vi "3_2_PTLF_Classification_Eval(FPGA)(PXI,sbRIO_Remote).vi"() -> ()   [LabVIEW 2020]
doc: "This example demonstrates the usage of \"Deep Neural Network Accelerator for FPGA\" for Face detection and running for inference on RT targets using FPGA."
uses:
  <vilib>/userDefined/High Color/nirio_resource_hc.ctl
  4973630c-52a8-4b5a-885b-d0de098afee9.vi
  0a2e89f5-e3e7-4dda-8136-2185c3411736.vi
  <vilib>/Ngene/Deep Learning Toolkit/Toolkit/NN_Data/subVIs/Get_Data_Vals/2D/NN_Data_Get_ValByRef(2D_SGL).vi
  <vilib>/Ngene/Deep Learning Toolkit/Toolkit/NN_Data/subVIs/Dataset/NN_Variant_to_DVR/2D/NN_Data_Variant_to_DVR(2D_SGL).vi
  <vilib>/FPGAPlugInAG/Dynamic/niLvFpga_Download_Dynamic.vi
  <vilib>/FPGAPlugInAG/Dynamic/niLvFpga_Run_Dynamic.vi
  <vilib>/Ngene/Deep Learning Toolkit/Toolkit/NN_Data/subVIs/Get_Data_Vals/2D/NN_Data_Get_ValByRef(2D_SGL_idx).vi
  <vilib>/Ngene/DeepLTK FPGA Addon/Toolkit/NNF_Host/API/NNF_Set_Input/NNF_Set_Input(1D_I8).vi
  <vilib>/Ngene/Deep Learning Toolkit/Toolkit/NN_Train/Eval_Loss/NN_Eval_Test_Error_Loss/NN_Eval(In1D_Out1D).vi
  <vilib>/Ngene/Deep Learning Toolkit/Toolkit/NN_Train/Eval_Loss/NN_Calc_Cofusion_Matrix/NN_Calc_Confusion_Matrix(In1D_Out1D).vi
  <vilib>/FPGAPlugInAG/Dynamic/niLvFpga_Close_Dynamic.vi
  <vilib>/rvi/interface/nirviMethod/nirviMethod.xnode
  <vilib>/rvi/interface/nirviCloseFPGA/nirviCloseFPGA.xnode
  <vilib>/Ngene/Deep Learning Toolkit/Toolkit/Deep_Learning_Toolkit_by_Ngene.lvlib
  <vilib>/Ngene/DeepLTK FPGA Addon/Toolkit/DeepLTK_FPGA_Addon.lvlib
  <vilib>/ptbypt/NI_PtbyPt.lvlib
panel:
  out "Dataset Size":i32=1200
  in  "FPGA Bitfile":path=path "D:/Ngene/GitHub/deepltk_fpga_examples/FPGA Bitfiles/NNF_sbRIO_9609_8Cores_120MHz.lvbitx"
  in  "FPGA target":T1="rio://10.0.0.39/RIO0" caption="RIO Device"
  out "Loop time(s)":dbl=12.583108442776332 format="%#_4p"
  out "Inference time(s)":dbl=0.07947161899999969 format="%#_4p"
  in  "Stop":bool
  out "Iterations":i32=1199
  in  "Dataset":path=path "D:/Ngene/GitHub/deepltk_fpga_examples/3_PTLF_Classification(PXI,sbRIO)/Dataset/Test"
  in  "Force CPU(All)?":bool
  out "GT":string="Swell"
  out "Pred":string="Sag"
  in  "index":i32=5
  out "Incorectly Classified Sample":sgl[](graph)=[-0.499, -0.502, -0.505, -0.507, -0.509, -0.51, -0.511, -0.512, -0.512, -0.512, -0.511, -0.51, -0.508, -0.506, -0.504, -0.501, -0.498, -0.495, -0.491, -0.487, -0.482, -0.477, -0.471, -0.466, -0.459, -0.453, -0.446, -0.439, -0.431, -0.423, -0.415, -0.406, -0.397, -0.388, -0.378, -0.368, -0.358, -0.347, -0.336, -0.325, -0.314, -0.303, -0.291, -0.279, -0.266, -0.254, -0.241, -0.228, -0.215, -0.202, -0.189, -0.175, -0.161, -0.148, -0.134, -0.12, -0.105, -0.091, -0.077, -0.062, -0.048, -0.034, -0.019, -0.005, 0.01, 0.024, 0.039, 0.053, 0.068, 0.082, 0.096, 0.111, 0.125, 0.139, 0.153, 0.166, 0.18, 0.193, 0.207, 0.22, 0.233, 0.246, 0.258, 0.271, 0.283, 0.295, 0.307, 0.318, 0.329, 0.34, 0.351, 0.362, 0.372, 0.381, 0.391, 0.4, 0.409, 0.418, 0.426, 0.434, 0.441, 0.448, 0.455, 0.462, 0.468, 0.473, 0.479, 0.484, 0.488, 0.492, 0.496, 0.5, 0.502, 0.505, 0.507, 0.509, 0.51, 0.511, 0.512, 0.512, 0.512, 0.511, 0.51, 0.508, 0.506, 0.504, 0.501, 0.498, 0.494, 0.49, 0.486, 0.481, 0.476, 0.471, 0.465, 0.459, 0.452, 0.445, 0.438, 0.43, 0.422, 0.414, 0.405, 0.396, 0.386, 0.377, 0.367, 0.357, 0.346, 0.335, 0.324, 0.313, 0.301, 0.289, 0.277, 0.265, 0.252, 0.24, 0.227, 0.214, 0.2, 0.187, 0.173, 0.16, 0.146, 0.132, 0.118, 0.104, 0.089, 0.075, 0.061, 0.046, 0.032, 0.017, 0.003, -0.012, -0.026, -0.041, -0.055, -0.069, -0.084, -0.098, -0.112, -0.126, -0.14, -0.154, -0.168, -0.182, -0.195, -0.208, -0.222, -0.235, -0.247, -0.26, -0.272, -0.284, -0.296, -0.308, -0.32, -0.331, -0.342, -0.352, -0.363, -0.373, -0.383, -0.392, -0.401, -0.41, -0.419, -0.427, -0.435, -0.442, -0.449, -0.456, -0.462, -0.468, -0.474, -0.479, -0.484, -0.489, -0.493, -0.497, -0.5, -0.503, -0.505, -0.507, -0.509, -0.51, -0.511, -0.512, -0.512, -0.511, -0.511, -0.51, -0.508, -0.506, -0.504, -0.501, -0.498, -0.494, -0.49, -0.486, -0.481, -0.476, -0.47, -0.464, -0.458, -0.451, -0.444, -0.437, -0.429, -0.421, -0.413, -0.404, -0.395, -0.385, -0.376, -0.366, -0.355, -0.345, -0.334, -0.323, -0.311, -0.3, -0.288, -0.276, -0.263, -0.251, -0.238, -0.225, -0.212, -0.199, -0.185, -0.172, -0.158, -0.144, -0.13, -0.116, -0.102, -0.088, -0.073, -0.059, -0.045, -0.03, -0.016, -0.001, 0.013, 0.028, 0.042, 0.057, 0.071, 0.085, 0.1, 0.114, 0.128, 0.142, 0.156, 0.17, 0.183, 0.197, 0.21, 0.223, 0.236, 0.249, 0.261, 0.274, 0.286, 0.298, 0.309, 0.321, 0.332, 0.343, 0.354, 0.364, 0.374, 0.384, 0.393, 0.402, 0.411, 0.42, 0.428, 0.436, 0.443, 0.45, 0.457, 0.463, 0.469, 0.475, 0.48, 0.485, 0.489, 0.493, 0.497, 0.5, 0.503, 0.506, 0.508, 0.509, 0.511, 0.511, 0.512, 0.512, 0.511, 0.511, 0.509, 0.508, 0.506, 0.503, 0.5, 0.497, 0.493, 0.489, 0.485, 0.48, 0.475, 0.469, 0.463, 0.457, 0.45, 0.443, 0.436, 0.428, 0.42, 0.412, 0.403, 0.394, 0.384, 0.374, 0.364, 0.354, 0.343, 0.333, 0.321, 0.31, 0.298, 0.286, 0.274, 0.262, 0.249, 0.237, 0.224, 0.211, 0.197, 0.184, 0.17, 0.156, 0.143, 0.129, 0.115, 0.1, 0.086, 0.072, 0.057, 0.043, 0.028, 0.014, -0.001, -0.015, -0.029, -0.044, -0.058, -0.073, -0.087, -0.101, -0.116, -0.13, -0.144, -0.157, -0.171, -0.185, -0.198, -0.211, -0.225, -0.238, -0.25, -0.263, -0.275, -0.287, -0.299, -0.311, -0.322, -0.333, -0.344, -0.355, -0.365, -0.375, -0.385, -0.394, -0.403, -0.412, -0.421, -0.429, -0.436, -0.444, -0.451, -0.458, -0.464, -0.47, -0.475, -0.481, -0.485, -0.49, -0.494, -0.497, -0.501, -0.503, -0.506, -0.508, -0.509, -0.511, -0.511, -0.512, -0.512, -0.511, -0.51, -0.509, -0.508, -0.505, -0.503, -0.5, -0.497, -0.493, -0.489, -0.484, -0.48, -0.474, -0.469, -0.463, -0.456, -0.45, -0.442, -0.435, -0.427, -0.419, -0.41, -0.402, -0.393, -0.383, -0.373, -0.363, -0.353, -0.342, -0.331, -0.32, -0.309, -0.297, -0.285, -0.273, -0.261, -0.248, -0.235, -0.222, -0.209, -0.196, -0.182, -0.169, -0.155, -0.141, -0.127, -0.113, -0.099, -0.084, -0.07, -0.056, -0.041, -0.027, -0.012, 0.002, 0.017, 0.031, 0.046, 0.06, 0.074, 0.089, 0.103, 0.117, 0.131, 0.145, 0.159, 0.173, 0.186, 0.2, 0.213, 0.226, 0.239, 0.252, 0.264, 0.277, 0.289, 0.301, 0.312, 0.324, 0.335, 0.345, 0.356, 0.366, 0.376, 0.386, 0.395, 0.404, 0.413, 0.422, 0.43, 0.437, 0.445, 0.452, 0.458, 0.465, 0.47, 0.476, 0.481, 0.486, 0.49, 0.494, 0.498, 0.501, 0.504, 0.506, 0.508, 0.51, 0.511, 0.511, 0.512, 0.512, 0.511, 0.51, 0.509, 0.507, 0.505, 0.503, 0.5, 0.496, 0.493, 0.488, 0.484, 0.479, 0.474, 0.468, 0.462, 0.456, 0.449, 0.442, 0.434, 0.426, 0.418, 0.409, 0.401, 0.391, 0.382, 0.372, 0.362, 0.352, 0.341, 0.33, 0.319, 0.307, 0.296, 0.284, 0.271, 0.259, 0.246, 0.234, 0.221, 0.207, 0.194, 0.181, 0.167, 0.153, 0.139, 0.125, 0.111, 0.097, 0.083, 0.068, 0.054, 0.04, 0.025, 0.011, -0.004, -0.018, -0.033, -0.047, -0.062, -0.076, -0.09, -0.105, -0.119, -0.133, -0.147, -0.161, -0.174, -0.188, -0.201, -0.215, -0.228, -0.241, -0.253, -0.266, -0.278, -0.29, -0.302, -0.314, -0.325, -0.336, -0.347, -0.357, -0.368, -0.377, -0.387, -0.396, -0.405, -0.414, -0.422, -0.431, -0.438, -0.445, -0.452, -0.459, -0.465, -0.471, -0.477, -0.482, -0.486, -0.491, -0.495, -0.498, -0.501, -0.504, -0.506, -0.508, -0.51, -0.511, -0.512, -0.512, -0.512, -0.511, -0.51, -0.509, -0.507, -0.505, -0.502, -0.499, -0.496, -0.492, -0.488, -0.483, -0.478, -0.473, -0.467, -0.461, -0.455, -0.448, -0.441, -0.433, -0.425, -0.417, -0.408, -0.4, -0.39, -0.381, -0.371, -0.361, -0.35, -0.34, -0.329, -0.317, -0.306, -0.294, -0.282, -0.27, -0.258, -0.245, -0.232, -0.219, -0.206, -0.193, -0.179, -0.165, -0.152, -0.138, -0.124, -0.11, -0.095, -0.081, -0.067, -0.052, -0.038, -0.023, -0.009, 0.006, 0.02, 0.035, 0.049, 0.063, 0.078, 0.092, 0.106, 0.121, 0.135, 0.148, 0.162, 0.176, 0.19, 0.203, 0.216, 0.229, 0.242, 0.255, 0.267, 0.279, 0.292, 0.303, 0.315, 0.326, 0.337, 0.348, 0.359, 0.369, 0.379, 0.388, 0.398, 0.406, 0.415, 0.423, 0.431, 0.439, 0.446, 0.453, 0.46, 0.466, 0.472, 0.477, 0.482, 0.487, 0.491, 0.495, 0.499, 0.502, 0.504, 0.507, 0.508, 0.51, 0.511, 0.512, 0.512, 0.512, 0.511, 0.51, 0.509, 0.507, 0.505, 0.502, 0.499, 0.495, 0.492, 0.487, 0.483, 0.478, 0.472, 0.467, 0.46, 0.454, 0.447, 0.44, 0.432, 0.424, 0.416, 0.407, 0.398, 0.389, 0.38, 0.37, 0.36, 0.349, 0.338, 0.327, 0.316, 0.305, 0.293, 0.281, 0.269, 0.256, 0.243, 0.231, 0.218, 0.204, 0.191, 0.177, 0.164, 0.15, 0.136, 0.122, 0.108, 0.094, 0.079, 0.065, 0.051, 0.036, 0.022, 0.007, -0.007, -0.022, -0.036, -0.051, -0.065, -0.08, -0.094, -0.108, -0.122, -0.136, -0.15, -0.164, -0.178, -0.191, -0.204, -0.218, -0.231, -0.244, -0.256, -0.269, -0.281, -0.293, -0.305, -0.316, -0.328, -0.339, -0.349, -0.36, -0.37, -0.38, -0.389, -0.399, -0.408, -0.416, -0.424, -0.432, -0.44, -0.447, -0.454, -0.461, -0.467, -0.472, -0.478, -0.483, -0.487, -0.492, -0.496, -0.499, -0.502, -0.505, -0.507, -0.509, -0.51, -0.511, -0.512, -0.512, -0.512, -0.511, -0.51, -0.508, -0.507, -0.504, -0.502, -0.499, -0.495, -0.491, -0.487, -0.482, -0.477, -0.472, -0.466, -0.46, -0.453, -0.446, -0.439, -0.431, -0.423, -0.415, -0.406, -0.397, -0.388, -0.378, -0.369, -0.358, -0.348, -0.337, -0.326, -0.315, -0.303, -0.291, -0.279, -0.267, -0.255, -0.242, -0.229, -0.216, -0.203, -0.189, -0.176, -0.162, -0.148, -0.134, -0.12, -0.106, -0.092, -0.078, -0.063, -0.049, -0.034, -0.02, -0.005, 0.009, 0.024, 0.038, 0.052, 0.067, 0.081, 0.095, 0.11, 0.124, 0.138, 0.152, 0.166, 0.179, 0.193, 0.206, 0.219, 0.232, 0.245, 0.258, 0.27, 0.282, 0.294, 0.306, 0.318, 0.329, 0.34, 0.351, 0.361, 0.371, 0.381, 0.39, 0.4, 0.409, 0.417, 0.425, 0.433, 0.441, 0.448, 0.455, 0.461, 0.467, 0.473, 0.478, 0.483, 0.488, 0.492, 0.496, 0.499, 0.502, 0.505, 0.507, 0.509, 0.51, 0.511, 0.512, 0.512, 0.512, 0.511, 0.51, 0.508, 0.506, 0.504, 0.501, 0.498, 0.495, 0.491, 0.486, 0.482, 0.477, 0.471, 0.465, 0.459, 0.452, 0.445, 0.438, 0.43, 0.422, 0.414, 0.405, 0.396, 0.387, 0.377, 0.367, 0.357, 0.347, 0.336, 0.325, 0.313, 0.302, 0.29, 0.278, 0.266, 0.253, 0.24, 0.228, 0.214, 0.201, 0.188, 0.174, 0.161, 0.147, 0.133, 0.119, 0.105, 0.09, 0.076, 0.062, 0.047, 0.033, 0.018, 0.004, -0.011, -0.025, -0.04, -0.054, -0.069, -0.083, -0.097, -0.111, -0.125, -0.139, -0.153, -0.167, -0.181, -0.194, -0.208, -0.221, -0.234, -0.247, -0.259, -0.272, -0.284, -0.296, -0.307, -0.319, -0.33, -0.341, -0.352, -0.362, -0.372, -0.382, -0.392, -0.401, -0.41, -0.418, -0.426, -0.434, -0.442, -0.449, -0.456, -0.462, -0.468, -0.474, -0.479, -0.484, -0.488, -0.493, -0.496, -0.5, -0.503, -0.505, -0.507, -0.509, -0.51, -0.511, -0.512, -0.512, -0.511, -0.511, -0.51, -0.508, -0.506, -0.504, -0.501, -0.498, -0.494, -0.49, -0.486, -0.481, -0.476, -0.47, -0.464, -0.458, -0.452, -0.445, -0.437, -0.429, -0.421, -0.413, -0.404, -0.395, -0.386, -0.376, -0.366, -0.356, -0.345, -0.335, -0.323, -0.312, -0.3, -0.289, -0.276, -0.264, -0.252, -0.239, -0.226, -0.213, -0.2, -0.186, -0.173, -0.159, -0.145, -0.131, -0.117, -0.103, -0.089, -0.074, -0.06, -0.045, -0.031, -0.017, -0.002, 0.012, 0.027, 0.041, 0.056, 0.07, 0.085, 0.099, 0.113, 0.127, 0.141, 0.155, 0.169, 0.182, 0.196, 0.209, 0.222, 0.235, 0.248, 0.261, 0.273, 0.285, 0.297, 0.309, 0.32, 0.331, 0.342, 0.353, 0.363, 0.373, 0.383, 0.393, 0.402, 0.411, 0.419, 0.427, 0.435, 0.443, 0.45, 0.456, 0.463, 0.469, 0.474, 0.48, 0.485, 0.489, 0.493, 0.497, 0.5, 0.503, 0.505, 0.508, 0.509, 0.51, 0.511, 0.512, 0.512, 0.511, 0.511, 0.509, 0.508, 0.693, 0.69, 0.686, 0.682, 0.677, 0.671, 0.665, 0.659, 0.652, 0.644, 0.636, 0.627, 0.618, 0.608, 0.598, 0.588, 0.576, 0.565, 0.553, 0.54, 0.527, 0.514, 0.5, 0.486, 0.472, 0.457, 0.442, 0.426, 0.41, 0.394, 0.377, 0.36, 0.343, 0.325, 0.308, 0.29, 0.272, 0.253, 0.234, 0.216, 0.197, 0.177, 0.158, 0.139, 0.119, 0.1, 0.08, 0.06, 0.04, 0.02, 0.0, -0.019, -0.039, -0.059, -0.079, -0.099, -0.118, -0.138, -0.157, -0.177, -0.196, -0.215, -0.234, -0.252, -0.271, -0.289, -0.307, -0.325, -0.342, -0.359, -0.376, -0.393, -0.409, -0.425, -0.441, -0.456, -0.471, -0.486, -0.5, -0.514, -0.527, -0.54, -0.552, -0.564, -0.576, -0.587, -0.598, -0.608, -0.618, -0.627, -0.635, -0.644, -0.651, -0.658, -0.665, -0.671, -0.677, -0.682, -0.686, -0.69, -0.693, -0.696, -0.698, -0.7, -0.701, -0.702, -0.702, -0.701, -0.7, -0.698, -0.696, -0.693, -0.69, -0.686, -0.681, -0.676, -0.671, -0.665, -0.658, -0.651, -0.643, -0.635, -0.626, -0.617, -0.607, -0.597, -0.586, -0.575, -0.563, -0.551, -0.539, -0.526, -0.513, -0.499, -0.485, -0.47, -0.455, -0.44, -0.424, -0.408, -0.392, -0.375, -0.358, -0.341, -0.323, -0.306, -0.288, -0.269, -0.251, -0.232, -0.213, -0.194, -0.175, -0.156, -0.136, -0.117, -0.097, -0.077, -0.058, -0.038, -0.018, 0.002, 0.022, 0.042, 0.061, 0.081, 0.101, 0.121, 0.14, 0.16, 0.179, 0.198, 0.217, 0.236, 0.254, 0.273, 0.291, 0.309, 0.327, 0.344, 0.361, 0.378, 0.395, 0.411, 0.427, 0.443, 0.458, 0.473, 0.487, 0.501, 0.515, 0.528, 0.541, 0.554, 0.566, 0.577, 0.588, 0.599, 0.609, 0.619, 0.628, 0.464, 0.47, 0.476, 0.481, 0.486, 0.49, 0.494, 0.498, 0.501, 0.504, 0.506, 0.508, 0.51, 0.511, 0.511, 0.512, 0.512, 0.511, 0.51, 0.509, 0.507, 0.505, 0.503, 0.5, 0.497, 0.493, 0.489, 0.484, 0.479, 0.474, 0.468, 0.462, 0.456, 0.449, 0.442, 0.435, 0.427, 0.418, 0.41, 0.401, 0.392, 0.382, 0.373, 0.363, 0.352, 0.342, 0.331, 0.319, 0.308, 0.296, 0.284, 0.272, 0.26, 0.247, 0.234, 0.221, 0.208, 0.195, 0.181, 0.168, 0.154, 0.14, 0.126, 0.112, 0.098, 0.084, 0.069, 0.055, 0.04, 0.026, 0.011, -0.003, -0.018, -0.032, -0.047, -0.061, -0.075, -0.09, -0.104, -0.118, -0.132, -0.146, -0.16, -0.174, -0.187, -0.201, -0.214, -0.227, -0.24, -0.253, -0.265, -0.277, -0.289, -0.301, -0.313, -0.324, -0.335, -0.346, -0.357, -0.367, -0.377, -0.387, -0.396, -0.405, -0.414, -0.422, -0.43, -0.438, -0.445, -0.452, -0.459, -0.465, -0.471, -0.476, -0.481, -0.486, -0.49, -0.494, -0.498, -0.501, -0.504, -0.506, -0.508, -0.51, -0.511, -0.512, -0.512, -0.512, -0.511, -0.51, -0.509, -0.507, -0.505, -0.502, -0.499, -0.496, -0.492, -0.488, -0.484, -0.479, -0.473, -0.468, -0.462, -0.455, -0.448, -0.441, -0.434, -0.426, -0.417, -0.409, -0.4, -0.391, -0.381, -0.372, -0.361, -0.351, -0.34, -0.329, -0.318, -0.307, -0.295, -0.283, -0.271, -0.258, -0.246, -0.233, -0.22, -0.207, -0.193, -0.18, -0.166, -0.152, -0.138, -0.124, -0.11, -0.096, -0.082, -0.068, -0.053, -0.039, -0.024, -0.01, 0.005, 0.019, 0.034, 0.048, 0.063, 0.077, 0.091, 0.106, 0.12, 0.134, 0.148, 0.162, 0.175, 0.189, 0.202, 0.215, 0.228, 0.241, 0.254, 0.267, 0.279, 0.291, 0.303, 0.314, 0.326, 0.337, 0.347, 0.358, 0.368, 0.378, 0.388, 0.397, 0.406, 0.415, 0.423, 0.431, 0.439, 0.446, 0.453, 0.459, 0.466, 0.471, 0.477, 0.482, 0.487, 0.491, 0.495, 0.498, 0.501, 0.504, 0.506, 0.508, 0.51, 0.511, 0.512, 0.512, 0.512, 0.511, 0.51, 0.509, 0.507, 0.505, 0.502, 0.499, 0.496, 0.492, 0.488, 0.483, 0.478, 0.473, 0.467, 0.461, 0.454, 0.447, 0.44, 0.433, 0.425, 0.417, 0.408, 0.399, 0.39, 0.38, 0.37, 0.36, 0.35, 0.339, 0.328, 0.317, 0.305, 0.293, 0.281, 0.269, 0.257, 0.244, 0.231, 0.218, 0.205, 0.192, 0.178, 0.165, 0.151, 0.137, 0.123, 0.109, 0.094, 0.08, 0.066, 0.051, 0.037, 0.022, 0.008, -0.007, -0.021, -0.035, -0.05, -0.064, -0.079, -0.093, -0.107, -0.121, -0.135, -0.149, -0.163, -0.177, -0.19, -0.204, -0.217, -0.23, -0.243, -0.256, -0.268, -0.28, -0.292, -0.304, -0.316, -0.327, -0.338, -0.349, -0.359, -0.369, -0.379, -0.389, -0.398, -0.407, -0.416, -0.424, -0.432, -0.44, -0.447, -0.454, -0.46, -0.466, -0.472, -0.478, -0.483, -0.487, -0.491, -0.495, -0.499, -0.502, -0.504, -0.507, -0.509, -0.51, -0.511, -0.512, -0.512, -0.512, -0.511, -0.51, -0.509, -0.507, -0.504, -0.502, -0.499, -0.495, -0.491, -0.487, -0.482, -0.477, -0.472, -0.466, -0.46, -0.454, -0.447, -0.439, -0.432, -0.424, -0.416, -0.407, -0.398, -0.389, -0.379, -0.369, -0.359, -0.348, -0.338, -0.327, -0.315, -0.304, -0.292, -0.28, -0.268, -0.255, -0.243, -0.23, -0.217, -0.204, -0.19, -0.177, -0.163, -0.149, -0.135, -0.121, -0.107, -0.093, -0.078, -0.064, -0.05, -0.035, -0.021, -0.006, 0.008, 0.023, 0.037, 0.052, 0.066, 0.08, 0.095, 0.109, 0.123, 0.137, 0.151, 0.165, 0.178, 0.192, 0.205, 0.219, 0.232, 0.244, 0.257, 0.269, 0.282, 0.294, 0.305, 0.317, 0.328, 0.339, 0.35, 0.36, 0.37, 0.38, 0.39, 0.399, 0.408, 0.417, 0.425, 0.433, 0.44, 0.448, 0.454, 0.461, 0.467, 0.473, 0.478, 0.483, 0.488, 0.492, 0.496, 0.499, 0.502, 0.505, 0.507, 0.509, 0.51, 0.511, 0.512, 0.512, 0.512, 0.511, 0.51, 0.508, 0.506, 0.504, 0.501, 0.498, 0.495, 0.491, 0.487, 0.482, 0.477, 0.471, 0.466, 0.459, 0.453, 0.446, 0.439, 0.431, 0.423, 0.415, 0.406, 0.397, 0.388, 0.378, 0.368, 0.358, 0.347, 0.336, 0.325, 0.314, 0.302, 0.291, 0.279, 0.266, 0.254, 0.241, 0.228, 0.215, 0.202, 0.189, 0.175, 0.161, 0.147, 0.134, 0.119, 0.105, 0.091, 0.077, 0.062, 0.048, 0.034, 0.019, 0.005, -0.01, -0.024, -0.039, -0.053, -0.068, -0.082, -0.096, -0.111, -0.125, -0.139, -0.153, -0.166, -0.18, -0.194, -0.207, -0.22, -0.233, -0.246, -0.258, -0.271, -0.283, -0.295, -0.307, -0.318, -0.329, -0.34, -0.351, -0.362, -0.372, -0.381, -0.391, -0.4, -0.409, -0.418, -0.426, -0.434, -0.441, -0.448, -0.455, -0.462, -0.468, -0.473, -0.479, -0.484, -0.488, -0.492, -0.496, -0.5, -0.502, -0.505, -0.507]
  out "Confusion Matrix (Table)":string[][](table)=[["200", "0", "0", "0", "0", "0", "1.0000"], ["0", "199", "0", "1", "0", "0", "0.9950"], ["0", "0", "200", "0", "0", "0", "1.0000"], ["0", "0", "0", "200", "0", "0", "1.0000"], ["0", "0", "1", "18", "181", "0", "0.9050"], ["0", "0", "2", "2", "3", "193", "0.9650"], ["1.0000", "1.0000", "0.9852", "0.9050", "0.9837", "1.0000", ""]]
  out "Error":sgl=0.0225
  out "Loss":sgl=0.029398046
  in  "Weight File Path":path=path "D:/Ngene/GitHub/deepltk_fpga_examples/3_PTLF_Classification(PXI,sbRIO)/Models/1_PTLF_Classification_Converted/NNF_ptlf_classifier_weights_24_11_21__13_54_07.bin"
  in  "Configuration File Path":path=path "D:/Ngene/GitHub/deepltk_fpga_examples/3_PTLF_Classification(PXI,sbRIO)/Models/1_PTLF_Classification_Converted/NNF_ptlf_classifier_net_cfg_24_11_21__13_54_07.cfg"
  in  "Scalers File Path":path=path "D:/Ngene/GitHub/deepltk_fpga_examples/3_PTLF_Classification(PXI,sbRIO)/Models/1_PTLF_Classification_Converted/NNF_ptlf_classifier_net_scalers_24_11_21__13_54_07.cfg"
  # "Overview: This VI is designed to evaluate (measure the accuracy of) the model when executed on FPGA in PXI systems.\nThis VI can also be used to run the evaluation on sbRIO Targets remotely (from Windows based PC)\nRequirements: \n• DeepLTK - Deep Learning Toolkit for LabVIEW (https://www.ngene.co/deep-learning-toolkit-for-labview)\n• DeepLTK FPGA Addon (https://www.ngene.co/deepltk-accelerator-for-fpga)\nInstructions:\n1. Select FPGA target at FPGA Target control. PXI or remote sbRIO FPGA target can be specified.\n2. Provide path to compiled FPGA bitfile at FPGA Bitfile control. A sample is available in the \"Examples\\FPGA Bitfiles\" folder. \n3. Provide the path to the dataset to be evaluated at Dataset.\n4. Provide paths to .cfg, .bin and scalers.cfg files generated during model conversion or sample from project (locted in \"Models\\1_PTLF_Classification_Converted\" folder ) at Network Configuration File Path, Weight File Path and Scalers File Path controls.\n5. Run the VI with the default remaining settings.\n6. Observe mersured accuracy at Loss, Error and Confusion Matrix indicators, and analyze Incorectly Classified Sample by selecting samples with help of index control.\n7. Press the Stop button to stop the VI.\n8. To measure reference accuracy (when executed on CPU) run 3_1_PTLF_Classification_Eval(CPU).vi located in the project.\nMore Examples: https://github.com/ngenehub/deepltk_fpga_examples"
  # "Copy resource path from NI MAX if needed"
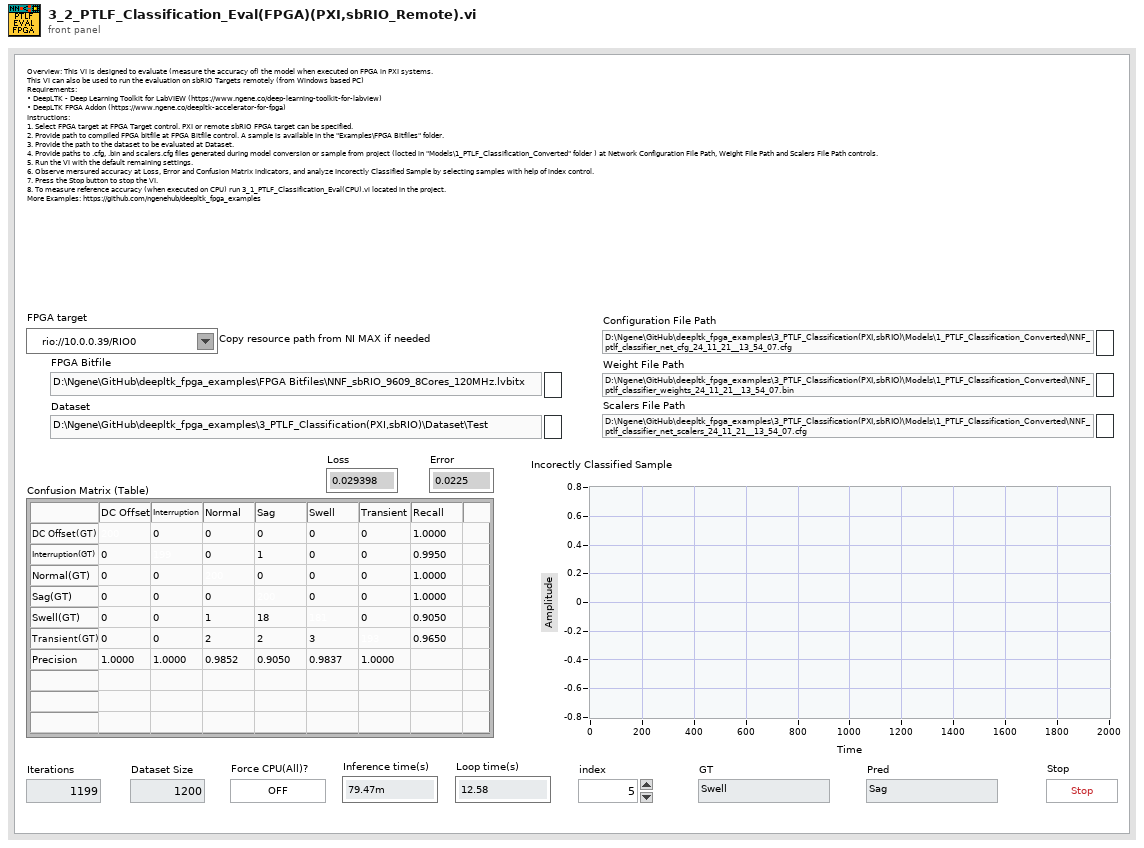
[diagram p1: front panel]
types:
  T1 = typedef "nirio_resource_hc.ctl" = tag
  T2 = typedef "Deep_Learning_Toolkit_by_Ngene.lvlib/NN_DataSets_All(In1D_Out1D).ctl" = cluster{"Train":T3, "Validation":T3, "Test":T3}
  T3 = typedef "Deep_Learning_Toolkit_by_Ngene.lvlib/NN_DataSet(In1D_Out1D).ctl" = cluster{"Inputs Ref.":variant, "Outputs Ref.":T4, "Dims_In":i32, "Dataset_Size":i32, "Dims_Out":i32, "Labels":string[], "File Paths":path[]}
  T4 = typedef "Deep_Learning_Toolkit_by_Ngene.lvlib/NN_Data_ref(2D_SGL).ctl" = refnum<data-value>
  T5 = typedef "DeepLTK_FPGA_Addon.lvlib/NNF.ctl" = cluster{"FPGA VI Ref ":refnum<k20>, "Subnets":T6[], "Dims_In":T8, "#Cores(enum)":T9, "NN_Ref":T10}
  T6 = typedef "DeepLTK_FPGA_Addon.lvlib/NNF_Subnet.ctl" = cluster{"Subnet Type":T7, "Subnet Data":variant, "Input Scaler":sgl, "Output Scaler":sgl}
  T7 = typedef "DeepLTK_FPGA_Addon.lvlib/NNF_Subnet_Type.ctl" = enum16{"CPU", "FPGA", "Split FPGA"}
  T8 = typedef "Deep_Learning_Toolkit_by_Ngene.lvlib/NN_Dims(C,H,W).ctl" = cluster{"C":i32, "H":i32, "W":i32}
  T9 = typedef "DeepLTK_FPGA_Addon.lvlib/NNF_No_Of_Cores.ctl" = enum16{"4CH", "8CH"}
  T10 = typedef "DeepLTK_FPGA_Addon.lvlib/NN_DVR.ctl" = refnum<data-value>
  T11 = typedef "Deep_Learning_Toolkit_by_Ngene.lvlib/NN_Layer.ctl" = cluster{"Name":string, "Layer_Data":variant, "Layer_Type":T12, "Dims_In":T8, "Layers_In":variant, "Dims_Out":T8, "Layers_Out":variant, "Metrics":T13, "GPU_Data":variant, "mBatch":i32, "NN_Device":T14, "NNg_hdls":T15, "Train?":bool, "Dimty":T16, "RecptField":T17}
  T12 = typedef "Deep_Learning_Toolkit_by_Ngene.lvlib/NN_Layer_Type.ctl" = enum16{"Input1D", "Input3D", "Conv1D", "Conv2D", "Conv2D_Adv", "MaxPool", "AvgPool", "UpSample", "DropOut3D", "ShortCut", "Concat", "SoftMax3D", "FC", "DropOut", "Softmax", "Flatten", "YOLO_v2", "YOLO_v4", "Activation", "BatchNormalization", "Unsupported"}
  T13 = typedef "Deep_Learning_Toolkit_by_Ngene.lvlib/NN_Layer_Metrics.ctl" = cluster{"Data":dbl, "Params":dbl, "Ops":dbl}
  T14 = typedef "Deep_Learning_Toolkit_by_Ngene.lvlib/NN_Device.ctl" = enum16{"CPU", "GPU"}
  T15 = typedef "Deep_Learning_Toolkit_by_Ngene.lvlib/nng_cuda_handles.ctl" = cluster{"cudnn":u64, "cublas":u64, "stream":u64, "curand":u64}
  T16 = typedef "Deep_Learning_Toolkit_by_Ngene.lvlib/NN_Layer_Dimty.ctl" = enum16{"1D", "3D"}
  T17 = typedef "Deep_Learning_Toolkit_by_Ngene.lvlib/NN_Layer_RF_State.ctl" = cluster{"Dims":T18, "J":T18}
  T18 = typedef "Deep_Learning_Toolkit_by_Ngene.lvlib/NN_Dims(V,H).ctl" = cluster{"V":i32, "H":i32}
  T19 = typedef "Deep_Learning_Toolkit_by_Ngene.lvlib/NN.ctl" = cluster{"Name":string, "No of Layers":i32, "mBatch":i32, "Layers":T20[], "Dimty":T21, "Dims_In":T8, "Dims_Out":T8, "Working_Dir":path, "Train?":bool, "Train_Params":T22, "LR_Update_Policy":T25, "Session Data":T27, "Ground_truth":T28, "NNg_hdls":T15, "NN_Device":T14, "GPU Id":i32, "Labels":string[], "Receptive Field":T18[], "Loss_Type":T29, "Loss_Cfg_Prms":variant, "NNG_WS":T30}
  T20 = typedef "Deep_Learning_Toolkit_by_Ngene.lvlib/NN_Layer_ref.ctl" = refnum<data-value>
  T21 = typedef "Deep_Learning_Toolkit_by_Ngene.lvlib/NN_In_Out_Dim-ty.ctl" = enum8{"In1D_Out1D", "In3D_Out1D", "In3D_Out3D", "In3D_OutBBox"}
  T22 = typedef "Deep_Learning_Toolkit_by_Ngene.lvlib/NN_Train_Params.ctl" = cluster{"Optimizer":T23, "Beta_1":sgl, "Beta_2":sgl, "Weight Decay(L1)":sgl, "Weight Decay(L2)":sgl, "Data_Sampling":T24}
  T23 = typedef "Deep_Learning_Toolkit_by_Ngene.lvlib/NN_Train_Optimizer.ctl" = enum16{"SGD", "Adam", "Adagrad", "Adadelta", "RMSProp", "Nesterov"}
  T24 = typedef "Deep_Learning_Toolkit_by_Ngene.lvlib/NN_Train_Data_Sampling.ctl" = enum16{"Random", "Sequential"}
  T25 = typedef "Deep_Learning_Toolkit_by_Ngene.lvlib/NN_LR_Policy_Cfg.ctl" = cluster{"Policy_Type":T26, "LR0":dbl, "k":sgl, "WarmUp_Policy":enum16{"Step", "Ramp"}, "WarmUp_Iter":i32, "WarmUp_Ratio":sgl}
  T26 = typedef "Deep_Learning_Toolkit_by_Ngene.lvlib/NN_LR_Policy_Type.ctl" = enum16{"Manual", "Step", "Exp", "1/t"}
  T27 = typedef "Deep_Learning_Toolkit_by_Ngene.lvlib/NN_Train_Session_Data.ctl" = cluster{"Epochs":sgl, "Tot_Iter":i32, "LR":sgl, "LR_iter":i32}
  T28 = typedef "Deep_Learning_Toolkit_by_Ngene.lvlib/NN_Ground_truth.ctl" = cluster{"Y":variant}
  T29 = typedef "Deep_Learning_Toolkit_by_Ngene.lvlib/NN_Loss_Type.ctl" = enum16{"None", "MSE", "CrossEntropy", "YOLO_v2", "YOLO_v4"}
  T30 = typedef "Deep_Learning_Toolkit_by_Ngene.lvlib/NNG_WS.ctl" = cluster{"NNG_WS_Mem":T31, "Max_WS_Size":i64}
  T31 = typedef "Deep_Learning_Toolkit_by_Ngene.lvlib/NNg_WS_Mem_DVR.ctl" = refnum<data-value>
  T32 = typedef "Deep_Learning_Toolkit_by_Ngene.lvlib/NN_Eval_Params.ctl" = cluster{"Loss":sgl, "Error":sgl}
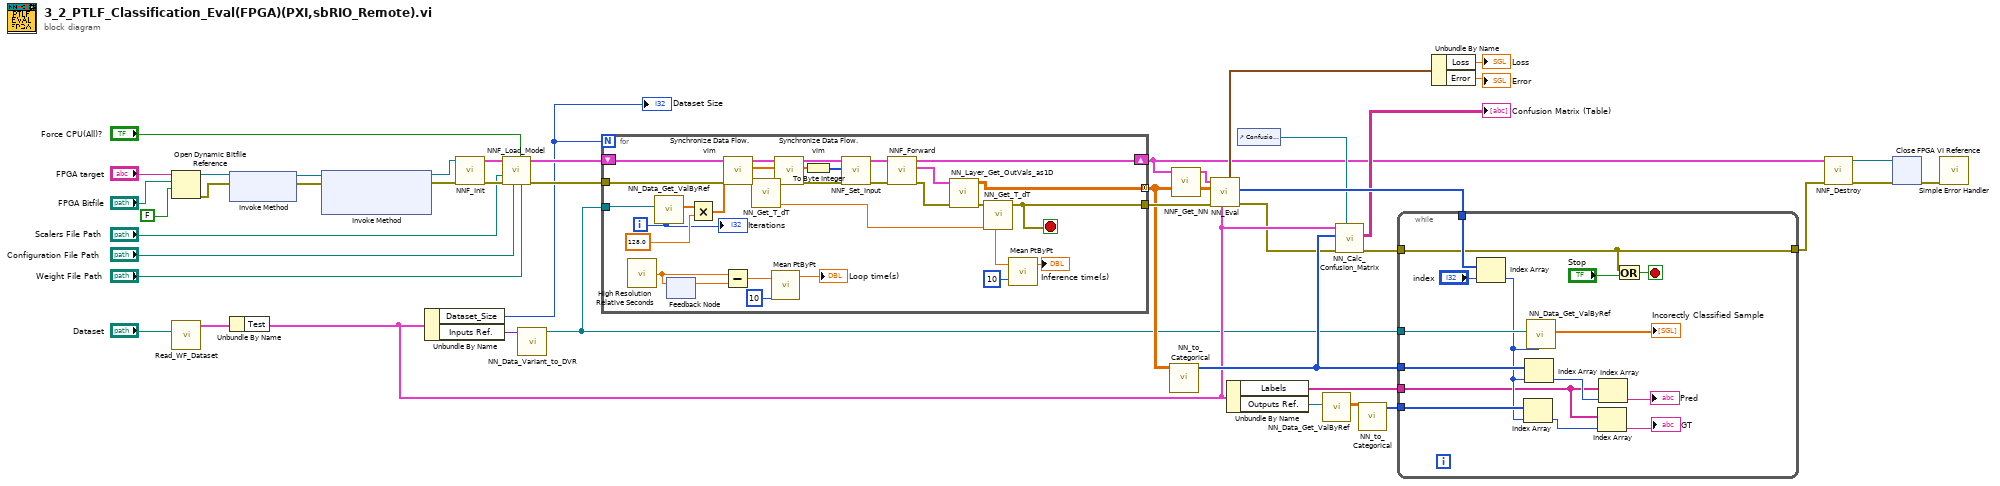
[diagram p0: block diagram]
diagram:
  n1 = Open Dynamic Bitfile Reference(0:"FPGA target", 1:"FPGA Bitfile", 2:FALSE ("Run When Loaded")) -> (5:w19:refnum<k20>, 8:w17:errorcluster)  [unwired: 2 in]
  n2 = call "Read_WF_Dataset.vi"("Test dataset path"="Dataset") -> ("NN_Dataset"=w21:T2)  [unwired: 10 in]
  n3 = xnode "Invoke Method"("FPGA VI Reference In"=w19, "error in"=w17) -> ("FPGA VI Reference Out"=w18:refnum<k20>, "error out"=w16:errorcluster)
  n4 = Unbundle By Name(w21) -> ("Test"=w15:T3)
  n5 = xnode "Invoke Method"("FPGA VI Reference In"=w18, "error in"=w16) -> ("FPGA VI Reference Out"=w22:refnum<k20>, "error out"=w41:errorcluster)  [unwired: 1 in]
  n6 = Unbundle By Name(w15) -> ("Dataset_Size"=w7:i32, "Inputs Ref."=w36:variant)
  "Dataset Size" <- w7
  n7 = call <vilib>:"NNF_Init.vi"("error in"=w41, "FPGA Interface"=w22) -> ("error out"=w44:errorcluster, "NNF out"=w43:T5)  [unwired: 7 in, 1 out]
  n8 = call <vilib>:"NNF_Load_Model.vi"("Weight File Path"="Weight File Path", "Force CPU(All)?"="Force CPU(All)?", "Network CFG File Path"="Configuration File Path", "Error in"=w44, "Scalers"="Scalers File Path", "NNF in"=w43) -> ("error Out"=w34:errorcluster, "NNF out"=w32:T5)  [unwired: 4 in]
  n9 = call-poly <vilib>:"NN_Data_Variant_to_DVR.vi"("Inputs Ref."=w36) -> ("DVR(2D_SGL)"=w2:T4)  [unwired: 9 in, 1 out]
  n10 = for {
    N: w7 -> [_]
    shift-right: [w76] -> w4
    shift-left: w32 -> [w61]
    tunnel: w2 -> [w75]
    tunnel: [w67] -> w27 mode=concatenating
    tunnel: [w51] -> w35
    tunnel: w34 -> [w60]
    i -> [w65]
    stop <- w51 stop-if-true
    n11 = call <vilib>:"High Resolution Relative Seconds.vi"() -> ("relative seconds"=w62:dbl)
    n12 = call-poly <vilib>:"NN_Data_Get_ValByRef.vi"("index (row)"=w65, "DVR(2D_SGL)"=w75) -> ("Value(1D_SGL)"=w74:sgl[])  [unwired: 6 in, 1 out]
    n13 = feedback #1() -> (w63:dbl)  [unwired: 1 in]
    n14 = feedback-in #1(w62) -> ()
    n15 = Multiply(x=w74, y=sgl 128.0 ("x")) -> (x*y=w58:sgl[])
    n16 = Subtract(x=w62, y=w63) -> (x-y=w64:dbl)
    n17 = call "Synchronize Data Flow.vim"("input 4"=w60, "input 2"=w58, "input 1"=w61) -> ("output 4"=w59:errorcluster, "output 2"=w55:sgl[], "output 1"=w57:T5)  [unwired: 1 in, 1 out]
    n18 = call <vilib>:"NN_Get_T_dT.vi"("error in (no error)"=w59) -> ("T_out"=w50:dbl, "error out"=w54:errorcluster)  [unwired: 6 in, 1 out]
    n19 = call <vilib>:"Mean PtByPt.vi"("x"=w64, "sample length"=10) -> ("mean"=→"Loop time(s)":dbl)  [unwired: 2 in, 1 out]
    n20 = call "Synchronize Data Flow.vim"("input 4"=w54, "input 2"=w55, "input 1"=w57) -> ("output 4"=w52:errorcluster, "output 2"=w53:sgl[], "output 1"=w56:T5)  [unwired: 1 in, 1 out]
    n21 = To Byte Integer(number=w53) -> (8bit integer=w66:i8[])
    n22 = call-poly <vilib>:"NNF_Set_Input.vi"("error in"=w52, "Data_in(1D_I8)"=w66, "NNF In"=w56) -> ("error out"=w71:errorcluster, "NNF out"=w72:T5)  [unwired: 7 in]
    n23 = call <vilib>:"NNF_Forward.vi"("error in"=w71, "NNF in"=w72) -> ("error out"=w69:errorcluster, "Last_Layer"=w70:T11, "NNF out"=w76:T5)  [unwired: 7 in]
    n24 = call <vilib>:"NN_Layer_Get_OutVals_as1D.vi"("error in (no error)"=w69, "Layer"=w70) -> ("error out"=w68:errorcluster, "Out(as1D)"=w67:sgl[][])  [unwired: 8 in]
    n25 = call <vilib>:"NN_Get_T_dT.vi"("T_in"=w50, "error in (no error)"=w68) -> ("error out"=w51:errorcluster, "dT"=w48:dbl)  [unwired: 5 in, 1 out]
    n26 = call <vilib>:"Mean PtByPt.vi"("x"=w48, "sample length"=10) -> ("mean"=→"Inference time(s)":dbl)  [unwired: 2 in, 1 out]
    "Iterations" <- w65
  }
  n27 = call <vilib>:"NN_to_Categorical.vi"("Prediction"=w27) -> ("Label_Idx"=w26:i32[])  [unwired: 10 in]
  n28 = call "NNF_Get_NN.vi"("NNF in"=w4) -> ("NN out"=w3:T19)  [unwired: 10 in]
  n29 = call-poly <vilib>:"NN_Eval.vi"("Dataset"=w15, "error in (no error)"=w35, "Predictions"=w27, "NN in"=w3) -> ("error out"=w10:errorcluster, "Incrct_Class_idx"=w28:i32[], "NN_Eval_Params"=w31:T32)  [unwired: 4 in, 1 out]
  n30 = Unbundle By Name(w15) -> ("Labels"=w1:string[], "Outputs Ref."=w14:T4)
  n31 = control-ref of="Confusion Matrix (Table)"() -> (w12:refnum<vi>)
  n32 = call-poly <vilib>:"NN_Data_Get_ValByRef.vi"("DVR(2D_SGL)"=w14) -> ("Value(2D_SGL)"=w25:sgl[][])  [unwired: 7 in, 1 out]
  n33 = call-poly <vilib>:"NN_Calc_Confusion_Matrix.vi"("Confusion Matrix (Table) ref."=w12, "error in (no error)"=w10, "Predictions"=w26, "Dataset"=w15) -> ("error out"=w9:errorcluster, "Confusion Matrix (Table)"=→"Confusion Matrix (Table)":string[][])  [unwired: 3 in, 3 out]
  n34 = call <vilib>:"NN_to_Categorical.vi"("Prediction"=w25) -> ("Label_Idx"=w24:i32[])  [unwired: 10 in]
  n35 = while {
    tunnel: w2 -> [w91]
    tunnel: w28 -> [w90]
    tunnel: w26 -> [w88]
    tunnel: w24 -> [w87]
    tunnel: [w79] -> w23
    tunnel: w9 -> [w79]
    tunnel: w1 -> [w77]
    stop <- w80 stop-if-true
    n36 = Index Array(array=w90, index="index") -> (element=w86:i32)
    n37 = Index Array(array=w87, index=w86) -> (element=w83:i32)
    n38 = Index Array(array=w88, index=w86) -> (element=w84:i32)
    n39 = call-poly <vilib>:"NN_Data_Get_ValByRef.vi"("index (row)"=w86, "DVR(2D_SGL)"=w91) -> ("Value(1D_SGL)"=→"Incorectly Classified Sample":sgl[])  [unwired: 6 in, 1 out]
    n40 = Index Array(array=w77, index=w83) -> (element=→"GT":string)
    n41 = Index Array(array=w77, index=w84) -> (element=→"Pred":string)
    n42 = Or(x=w79, y="Stop") -> (x .or. y?=w80:bool)
  }
  n43 = Unbundle By Name(w31) -> ("Loss"=→"Loss":sgl, "Error"=→"Error":sgl)
  n44 = call <vilib>:"NNF_Destroy.vi"("error in"=w23, "NNF in"=w4) -> ("error out"=w40:errorcluster, "FPGA VI Ref"=w39:refnum<k20>)  [unwired: 8 in]
  n45 = xnode "Close FPGA VI Reference"("FPGA VI Reference In"=w39, "error in"=w40) -> ("error out"=w38:errorcluster)
  n46 = call <vilib>:"Simple Error Handler.vi"("error in (no error)"=w38) -> ()  [unwired: 4 in, 5 out]
